vi "Process Test Record.vi"(8 "error in (no error)":errorcluster, 10 "Signal":string, 11 "TestRec":T1) -> (0 "error out":errorcluster, 3 "Data Record":T2)   [LabVIEW 2011]
uses:
  Controls/Test Data Record.ctl
  Controls/DVR of CSV Tests Data.ctl
  Controls/CSVs Tests Data.ctl
  Controls/Test Column Data.ctl
  Analysis/Read Actual Values From Log File.vi
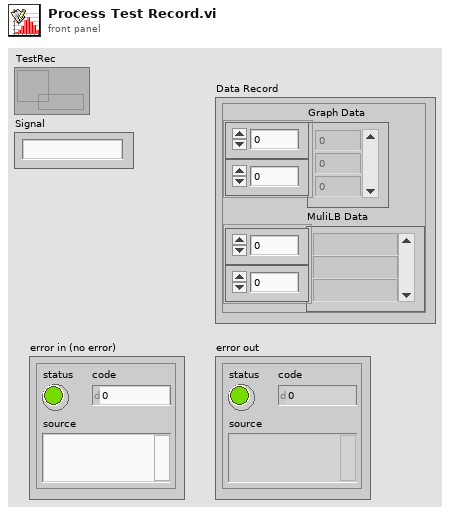
[diagram p1: front panel]
types:
  T1 = typedef "DVR of CSV Tests Data.ctl" = refnum<data-value>
  T2 = typedef "Test Data Record.ctl" = cluster{"Graph Data":dbl[][], "MuliLB Data":string[][]}
  T3 = typedef "CSVs Tests Data.ctl" = cluster{"Test Data":T4[], "CsvPath":path, "LogPath":path, "Pass?":bool, "Error":errorcluster}
  T4 = typedef "Test Column Data.ctl" = cluster{"Chn":string, "ExpVals":dbl[], "TimeStamps":i64[], "NegTol":dbl, "PosTol":dbl}
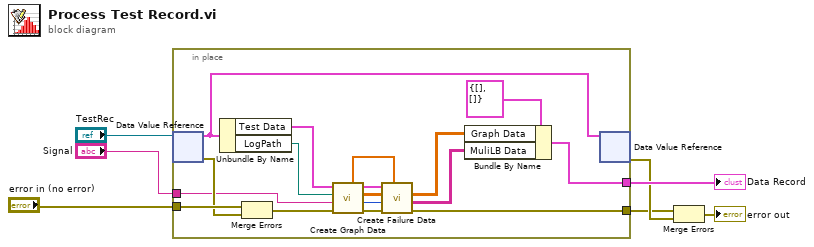
[diagram p0: block diagram]
diagram:
  n1 = in-place {
    in-place-border: "error in (no error)" -> [w24]
    in-place-border: "Signal" -> [w21]
    in-place-border: [w18] -> w7
    in-place-border: [w9] -> w3
    n2 = in-place-dvr #1("TestRec") -> (w20:T3, w22:errorcluster)
    n3 = Unbundle By Name(w20) -> ("Test Data"=w16:T4[], "LogPath"=w17:path)
    n4 = Merge Errors(w24, w22) -> (w23:errorcluster)
    n5 = call "Create Graph Data.vi"("error in (no error)"=w23, "Signal"=w21, "LogPath"=w17, "Test Data"=w16) -> ("error out"=w10:errorcluster, "Idx"=w11:i32, "Graph Data"=w15:dbl[][], "Test Data dup"=w14:T4[], "System Time"=w8:dbl[])  [unwired: 3 in]
    n6 = call "Create Failure Data.vi"("System Time"=w8, "error in (no error)"=w10, "Idx"=w11, "Graph Data"=w15, "Test Data"=w14) -> ("error out"=w9:errorcluster, "MultiLB Data"=w12:string[][], "Graph Data dup"=w13:dbl[][])  [unwired: 4 in]
    n7 = Bundle By Name(cluster=T2 {"Graph Data"=[], "MuliLB Data"=[]} ("Data Record"), "Graph Data"=w13, "MuliLB Data"=w12) -> (w18:T2)
    n8 = in-place-dvr #1(w20) -> (w5:errorcluster)  [unwired: 1 out]
  }
  "Data Record" <- w7
  n9 = Merge Errors(w3, w5) -> (→"error out":errorcluster)
